vi "AnnexDFilter.vi"(8 "error in (no error)":errorcluster, 10 "PmuConfig":T1={"Class"=enum."M", "Fs"=60, "F0"=60, "FSamp"=60, "SettlingTime"=0.0, "T0"=0.0}) -> (0 "error out":errorcluster, 1 "WindowType":string, 2 "FilterParams":dbl[](array[numeric]))   [LabVIEW 2014, in "SensorPlugins.lvlib" / "C37.118 Sim.lvclass"]
uses:
  C37.118 Sim.lvclass
  PmuBaseClass/Typedef/PmuConfig.ctl
  <vilib>/Utility/error.llb/Error Cluster From Error Code.vi
  <vilib>/ErrorRing/Error Ring.xnode
  PmuBaseClass/PmuBase.lvclass
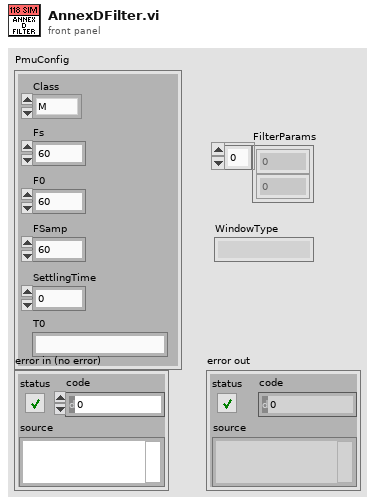
[diagram p1: front panel]
types:
  T1 = typedef "SensorPlugins.lvlib/PmuBase.lvclass/PmuConfig.ctl" = cluster{"Class":enum16{"M", "P"}, "Fs":i32, "F0":i32, "FSamp":i32, "SettlingTime":dbl, "T0":ext}
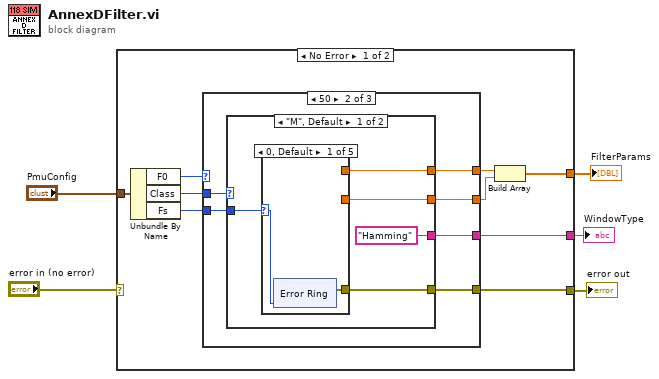
[diagram p0: block diagram]
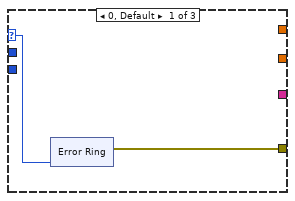
[diagram p2: hidden frame]
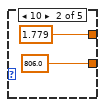
[diagram p3: hidden frame]
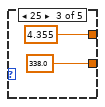
[diagram p4: hidden frame]
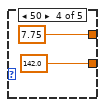
[diagram p5: hidden frame]
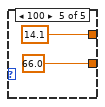
[diagram p6: hidden frame]
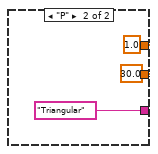
[diagram p7: hidden frame]
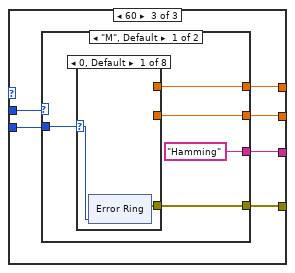
[diagram p8: hidden frame]
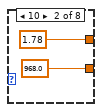
[diagram p9: hidden frame]
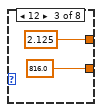
[diagram p10: hidden frame]
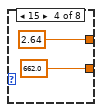
[diagram p11: hidden frame]
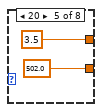
[diagram p12: hidden frame]
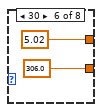
[diagram p13: hidden frame]
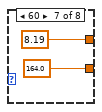
[diagram p14: hidden frame]
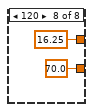
[diagram p15: hidden frame]
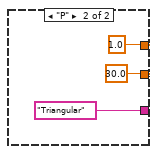
[diagram p16: hidden frame]
diagram:
  n1 = case shown="No Error" "error in (no error)" {
    selector: "error in (no error)" -> [_ w92]
    tunnel: "PmuConfig" -> [w14 _]
    tunnel: [w6 _] -> w4
    tunnel: [w8 _] -> w3
    tunnel: [w7 w92] -> w1
    frame No Error {
      n2 = Unbundle By Name(w14) -> ("F0"=w13:i32, "Class"=w12:enum16{"M", "P"}, "Fs"=w11:i32)
      n3 = case shown="50" w13 {
        selector: w13 -> [w15 _ _]
        tunnel: [w16 w25 w56] -> w7
        tunnel: w12 -> [_ w29 w60]
        tunnel: w11 -> [_ w28 w59]
        tunnel: [_ w27 w58] -> w10
        tunnel: [_ w26 w57] -> w9
        tunnel: [_ w24 w55] -> w8
        frame 0, Default {
          n4 = xnode "Error Ring"("parameter 0"=w15) -> ("error out"=w16:errorcluster)
        }
        frame 50 {
          n5 = case shown="\"M\", Default" w29 {
            tunnel: w28 -> [w34 _]
            tunnel: [w33 1.0] -> w27
            tunnel: [w32 30.0] -> w26
            tunnel: [w31 _] -> w25
            tunnel: ["Hamming" "Triangular"] -> w24
            frame "M", Default {
              n6 = case shown="0, Default" w34 {
                selector: w34 -> [w36 _ _ _ _]
                tunnel: [_ 1.779 4.355 7.75 14.1] -> w33
                tunnel: [_ 806.0 338.0 142.0 66.0] -> w32
                tunnel: [w35 _ _ _ _] -> w31
                frame 0, Default {
                  n7 = xnode "Error Ring"("parameter 0"=w36) -> ("error out"=w35:errorcluster)
                }
                frame 10 {
                }
                frame 25 {
                }
                frame 50 {
                }
                frame 100 {
                }
              }
            }
            frame "P" {
            }
          }
        }
        frame 60 {
          n8 = case shown="\"M\", Default" w60 {
            tunnel: w59 -> [w65 _]
            tunnel: [w64 1.0] -> w58
            tunnel: [w63 30.0] -> w57
            tunnel: [w62 _] -> w56
            tunnel: ["Hamming" "Triangular"] -> w55
            frame "M", Default {
              n9 = case shown="0, Default" w65 {
                selector: w65 -> [w67 _ _ _ _ _ _ _]
                tunnel: [_ 1.78 2.125 2.64 3.5 5.02 8.19 16.25] -> w64
                tunnel: [_ 968.0 816.0 662.0 502.0 306.0 164.0 70.0] -> w63
                tunnel: [w66 _ _ _ _ _ _ _] -> w62
                frame 0, Default {
                  n10 = xnode "Error Ring"("parameter 0"=w67) -> ("error out"=w66:errorcluster)
                }
                frame 10 {
                }
                frame 12 {
                }
                frame 15 {
                }
                frame 20 {
                }
                frame 30 {
                }
                frame 60 {
                }
                frame 120 {
                }
              }
            }
            frame "P" {
            }
          }
        }
      }
      n11 = Build Array(w10, w9) -> (w6:dbl[])
    }
    frame Error {
    }
  }
  "FilterParams" <- w4
  "WindowType" <- w3
  "error out" <- w1
